vi "ExSubWaitSpec.vi"(2 "error in (no error)":errorcluster, 3 "Spectrometer Handle":u32) -> (0 "error out":errorcluster, 1 "Spectrometer handle":u32)   [LabVIEW 2011]
panel:
  # "ExSubWaitSpec:\nThis Sub-VI waits for a spectograph\noperation to complete."
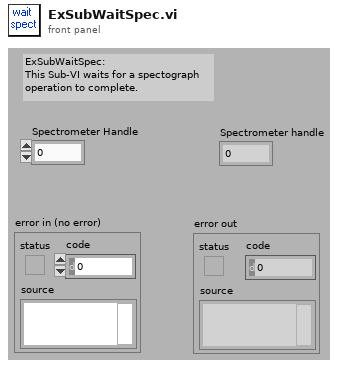
[diagram p1: front panel]
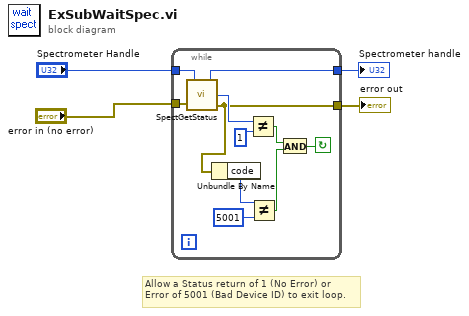
[diagram p0: block diagram]
diagram:
  # "Allow a Status return of 1 (No Error) or\nError of 5001 (Bad Device ID) to exit loop."
  n1 = while {
    tunnel: "Spectrometer Handle" -> [w15]
    tunnel: "error in (no error)" -> [w14]
    tunnel: [w13] -> w1
    tunnel: [w6] -> w2
    stop <- w8 continue-if-true
    n2 = call <userlib>:"SpectGetStatus.vi"("Spectrometer Handle"=w15, "error in"=w14) -> ("Spectrometer Handle"=w13:u32, "Command Status"=w7:u32, "error out"=w6:errorcluster)
    n3 = Unbundle By Name(w6) -> ("code"=w5:i32)
    n4 = Not Equal?(x=w7, y=u32 1) -> (x != y?=w10:bool)
    n5 = Not Equal?(x=w5, y=5001) -> (x != y?=w9:bool)
    n6 = And(x=w10, y=w9) -> (x .and. y?=w8:bool)
  }
  "error out" <- w2
  "Spectrometer handle" <- w1
